vi "Unreserve Device.vi"(8 "error in (no error)":errorcluster, 11 "SLSC Switch in":refnum<class "SLSC Switch.lvclass">) -> (0 "error out":errorcluster, 3 "SLSC Switch out":refnum<class "SLSC Switch.lvclass">)   [LabVIEW 2015, in "SLSC Switch.lvclass"]
uses:
  SLSC Switch.lvclass
  SLSC Switch.lvclass/SLSC Switch.ctl
  <vilib>/SLSC/SLSC.lvlib
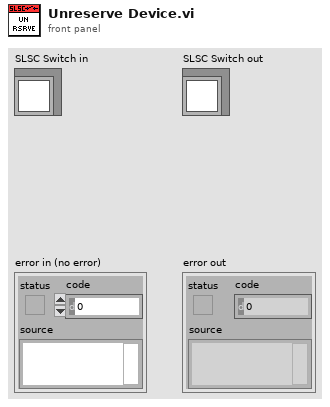
[diagram p1: front panel]
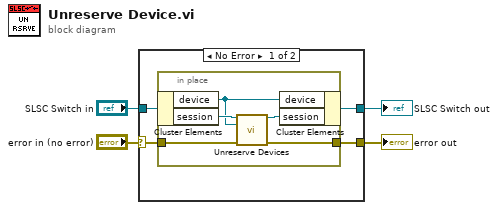
[diagram p0: block diagram]
diagram:
  n1 = case shown="No Error" "error in (no error)" {
    selector: "error in (no error)" -> [w5 w15]
    tunnel: [w8 w15] -> w3
    tunnel: [w7 w14] -> w1
    tunnel: "SLSC Switch in" -> [w6 w14]
    frame No Error {
      n2 = in-place {
        in-place-border: [w13] -> w8
        in-place-border: w5 -> [w12]
        n3 = in-place-cluster #1(w6) -> ("device"=w10:refnum<k21>, "session"=w11:refnum<k21>)
        n4 = call <vilib>:"Unreserve Devices.vi"("session in"=w11, "devices"=w10, "error in (no error)"=w12) -> ("session out"=w9:refnum<k21>, "error out"=w13:errorcluster)  [unwired: 11 in]
        n5 = in-place-cluster #1("device"=w10, "session"=w9) -> (w7:refnum<class "SLSC Switch.lvclass">)
      }
    }
    frame Error {
    }
  }
  "error out" <- w3
  "SLSC Switch out" <- w1
